vi "DS1820TEMP 2.vi"() -> ()   [LabVIEW 2017]
uses:
  <vilib>/LabVIEW Interface for Arduino/Type Defs/Pin Mode.ctl
  <vilib>/Instr/_visa.llb/VISA Configure Serial Port (Instr).vi
  <vilib>/LabVIEW Interface for Arduino/LabVIEW Interface for Arduino.lvlib
panel:
  in  "Lim_inf":dbl
  in  "Lim_sup":dbl
  in  "Stop":bool
  out "TEMP":string
  out "TEMP GAUGE":dbl(slide) scale=0.0..100.0
  out "WAVE TEMP":i32(graph)
  in  "stop":bool
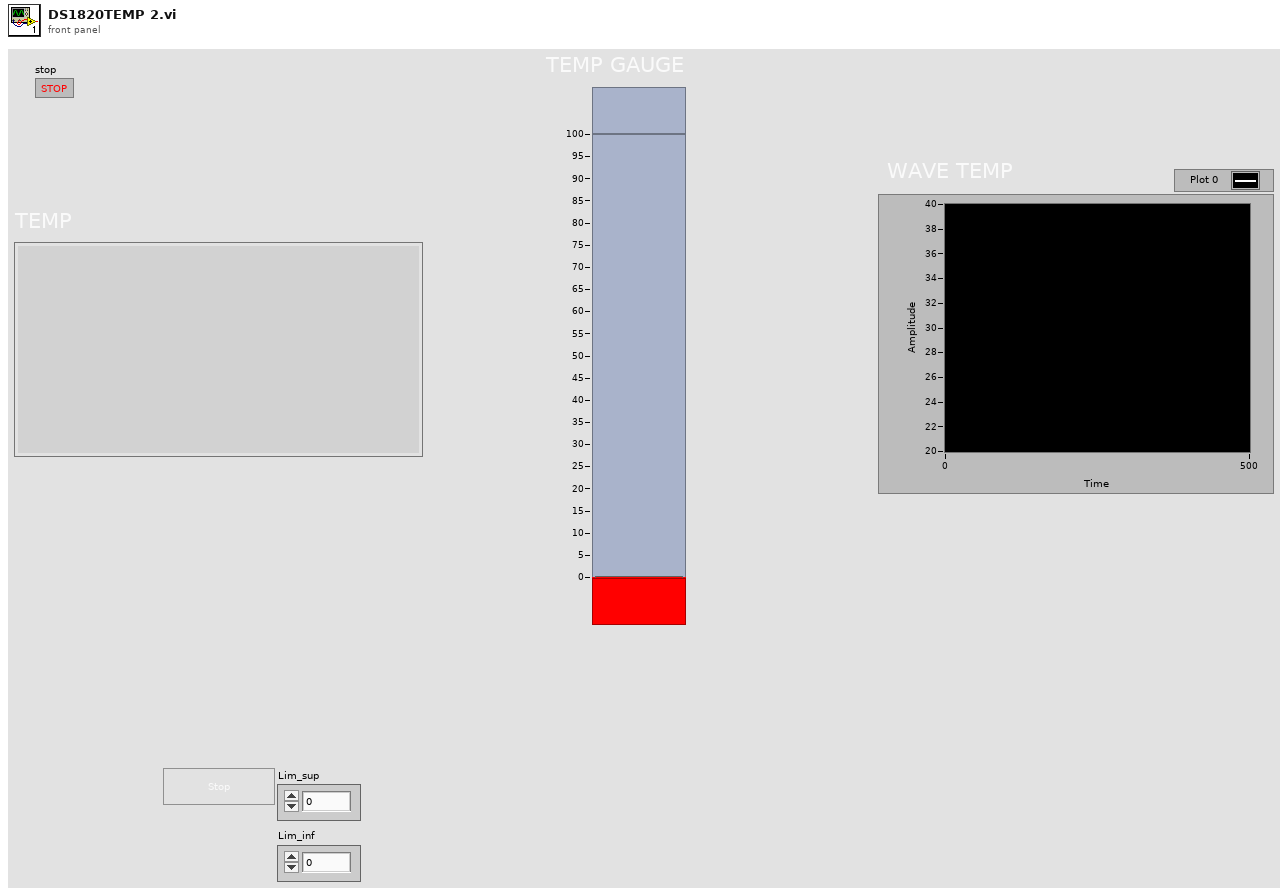
[diagram p1: front panel]
types:
  T1 = typedef "LabVIEW Interface for Arduino.lvlib/Pin Mode.ctl" = enum8{"Input", "Output"}
  T2 = typedef "LabVIEW Interface for Arduino.lvlib/Arduino Resource.ctl" = cluster{"VISA resource":refnum<visa-resource-name>, "Board Type":T3, "Connection Type":enum8{"USB / Serial"}, "Bytes Per Packet (15)":u8}
  T3 = typedef "LabVIEW Interface for Arduino.lvlib/Board Type.ctl" = enum16{"Uno", "Dimuelanove w/Atmega 328", "Mega 2560"}
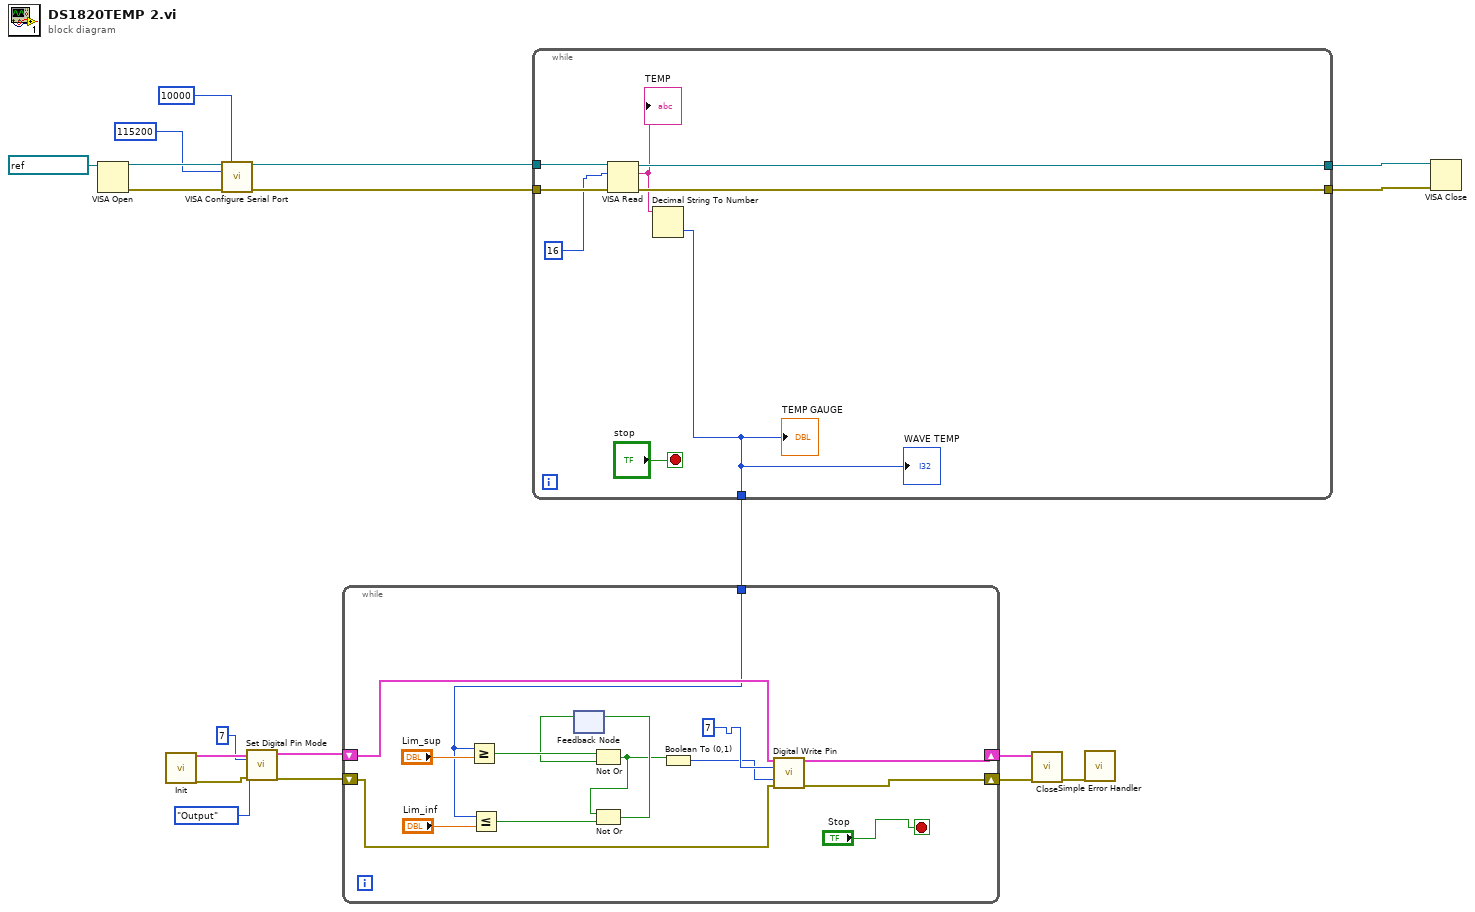
[diagram p0: block diagram]
diagram:
  n1 = VISA Open(VISA resource name=refnum<visa-resource-name> "COM3") -> (VISA resource name=w15:refnum<visa-resource-name>, error out=w14:errorcluster)  [unwired: 4 in]
  n2 = call <vilib>:"Init.vi"() -> ("Arduino Resource"=w5:T2, "error out"=w4:errorcluster)  [unwired: 18 in]
  n3 = call-poly "VISA Configure Serial Port"("VISA resource name"=w15, "timeout (10sec)"=u32 10000, "baud rate (9600)"=u32 115200, "error in (no error)"=w14) -> ("VISA resource name out"=w17:refnum<visa-resource-name>, "error out"=w16:errorcluster)  [unwired: 10 in]
  n4 = call <vilib>:"Set Digital Pin Mode.vi"("Arduino Resource"=w5, "Digital I/O Pin"=u8 7, "Pin Mode (Input)"=Pin_Mode."Output", "error in"=w4) -> ("Arduino Resource"=w7:T2, "error out"=w6:errorcluster)  [unwired: 10 in]
  n5 = while {
    tunnel: [w27] -> w19
    tunnel: [w26] -> w18
    tunnel: w17 -> [w25]
    tunnel: w16 -> [w24]
    tunnel: [w20] -> w1
    stop <- "stop" stop-if-true
    n6 = VISA Read(VISA resource name=w25, byte count=u32 16, error in (no error)=w24) -> (VISA resource name out=w27:refnum<visa-resource-name>, read buffer=w23:string, error out=w26:errorcluster)  [unwired: 1 out]
    "TEMP" <- w23
    n7 = Decimal String To Number(string=w23) -> (number=w20:i32)  [unwired: 2 in, 1 out]
    "TEMP GAUGE" <- w20
    "WAVE TEMP" <- w20
  }
  n8 = while {
    shift-right: [w42] -> w10
    shift-left: w7 -> [w30]
    shift-right: [w41] -> w9
    shift-left: w6 -> [w29]
    tunnel: w1 -> [w28]
    stop <- "Stop" stop-if-true
    n9 = Greater Or Equal?(x=w28, y="Lim_sup") -> (x >= y?=w37:bool)
    n10 = Less Or Equal?(x=w28, y="Lim_inf") -> (x <= y?=w38:bool)
    n11 = feedback #1() -> (w36:bool)  [unwired: 1 in]
    n12 = Not Or(1:w36, 2:w37) -> (0:w32:bool)
    n13 = Not Or(1:w38, 2:w32) -> (0:w35:bool)
    n14 = feedback-in #1(w35) -> ()
    n15 = Boolean To (0,1)(Boolean=w32) -> (0, 1=w31:i16)
    n16 = call <vilib>:"Digital Write Pin.vi"("Arduino Resource"=w30, "Digital I/O Pin (0)"=u8 7, "Value (0)"=w31, "error in"=w29) -> ("Arduino Resource"=w42:T2, "error out"=w41:errorcluster)  [unwired: 10 in]
  }
  n17 = call <vilib>:"Close.vi"("Arduino Resource"=w10, "error in"=w9) -> ("error out"=w8:errorcluster)  [unwired: 13 in]
  n18 = call <vilib>:"Simple Error Handler.vi"("error in (no error)"=w8) -> ()  [unwired: 4 in, 5 out]
  n19 = VISA Close(VISA resource name=w19, error in (no error)=w18) -> ()  [unwired: 1 out]
